vi "modifySALLVLibElementsForRT.vi"(10 "Path to VIs folder":path=path "C:/LSST_TS/SystemSW/ts_sallabviewrt_tools/ts_sallv_exa/VIs") -> ()   [LabVIEW 2016]
uses:
  VI/VI.lvclass
panel:
  out "error out":errorcluster
  in  "error in (no error)":errorcluster
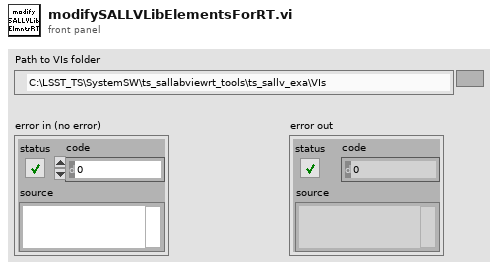
[diagram p1: front panel]
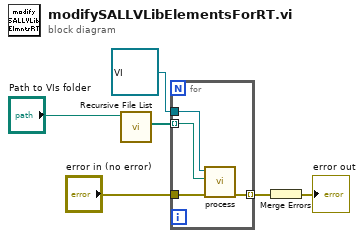
[diagram p0: block diagram]
diagram:
  n1 = call <vilib>:"Recursive File List.vi"("Folder Path"="Path to VIs folder") -> ("All Files in Dir"=w4:path[])  [unwired: 6 in, 4 out]
  n2 = for {
    tunnel: refnum<class "VI.lvclass"> refnum ("VI in") -> [w10]
    tunnel: w4 -> [w9] mode=indexing
    tunnel: "error in (no error)" -> [w8]
    tunnel: [w7] -> w2 mode=indexing
    n3 = call-dynamic "process.vi"("error in (no error)"=w8, "Path"=w9, "VI in"=w10) -> ("error out"=w7:errorcluster)  [unwired: 7 in, 1 out]
  }
  n4 = Merge Errors(w2) -> (→"error out":errorcluster)
